vi "Handle Last Ack Core.vi"(4 "error in (no error)":errorcluster, 6 "Last Ack":refnum<class "Last Ack.lvclass">, 7 "Application in":refnum<class "Application.lvclass">) -> (0 "error out":errorcluster, 3 "Application out":refnum<class "Application.lvclass">)   [LabVIEW 2022 SP3, in "Application.lvlib" / "Application.lvclass"]
doc: "(<B>Filename</B>: Actor Framework.lvlib:Actor.lvclass:Handle Last Ack Core.vi)\n\nDefines how the caller actor responds to the Last Ack message from a nested actor. The Last Ack message is the final message a nested actor sends to its caller before it shuts down. The message contains information about the final state of the nested actor.\n\nBy default, this method does nothing except return any error the nested actor sent. A descendant class may override this method to define behavior."
uses:
  Application.lvclass
  <vilib>/ActorFramework/LastAck/Last Ack.lvclass
  C:/Program Files/National Instruments/LabVIEW 2022/vi.lib/ActorFramework/Actor/Actor.lvclass
  <vilib>/ActorFramework/LastAck/Last Ack.lvclass/Last Ack.ctl
  <vilib>/ActorFramework/Actor/Actor.lvclass/Actor.ctl
  <vilib>/ActorFramework/Message Enqueuer/Message Enqueuer.lvclass/Message Enqueuer.ctl
  <vilib>/ActorFramework/Message Enqueuer/Init from Existing Queue.vi
  <vilib>/ActorFramework/Message Enqueuer/Enqueue.vi
  <vilib>/ActorFramework/Stop Msg/Stop Msg.lvclass
  C:/Program Files/National Instruments/LabVIEW 2022/vi.lib/ActorFramework/Message/Message.lvclass
  <vilib>/ActorFramework/Message Priority Queue/Priority Enqueue.vi
  <vilib>/ActorFramework/Message Enqueuer/Message Enqueuer.lvclass
  Application.lvclass/Application.ctl
  <vilib>/ActorFramework/Actor/Actor.lvclass
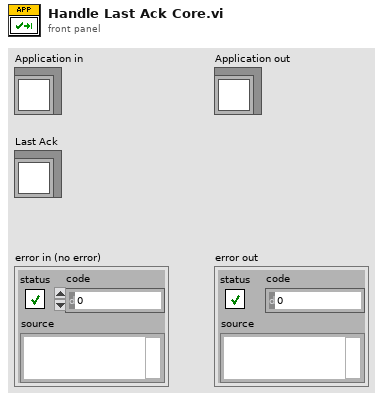
[diagram p1: front panel]
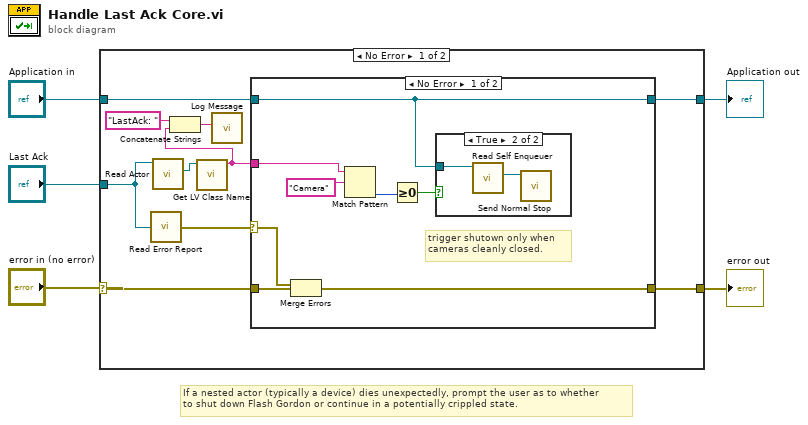
[diagram p0: block diagram]
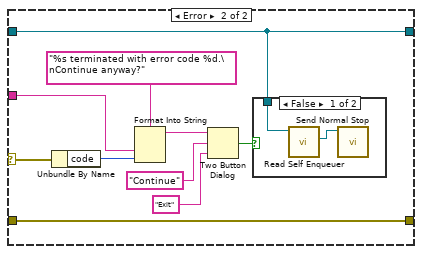
[diagram p3: hidden frame]
diagram:
  # "If a nested actor (typically a device) dies unexpectedly, prompt the user as to whether\nto shut down Flash Gordon or continue in a potentially crippled state."
  n1 = case shown="No Error" "error in (no error)" {
    selector: "error in (no error)" -> [w12 w38]
    tunnel: [w13 w38] -> w5
    tunnel: [w10 w39] -> w4
    tunnel: "Application in" -> [w11 w39]
    tunnel: "Last Ack" -> [w15 _]
    frame No Error {
      n2 = call <vilib>:"Read Error Report.vi"("Last Ack"=w15) -> ("error report"=w14:errorcluster)
      n3 = call <vilib>:"Read Actor.vi"("Last Ack"=w15) -> ("Actor"=w9:refnum<class "Actor.lvclass">)  [unwired: 10 in]
      n4 = call <vilib>:"Get LV Class Name.vi"("object"=w9) -> ("class name"=w7:string)  [unwired: 9 in, 1 out]
      n5 = Concatenate Strings("LastAck: " ("string"), w7) -> (w8:string)
      n6 = call "Log Message.vi"("input"=w8) -> ()  [unwired: 9 in, 2 out]
      n7 = case shown="No Error" w14 {
        selector: w14 -> [w17 w31]
        tunnel: [w16 w28] -> w13
        tunnel: w12 -> [w18 w28]
        tunnel: w11 -> [w20 w30]
        tunnel: [w20 w30] -> w10
        tunnel: w7 -> [w19 w26]
        frame No Error {
          # "trigger shutown only when\ncameras cleanly closed."
          n8 = Merge Errors(w17, w18) -> (w16:errorcluster)
          n9 = Match Pattern(string=w19, regular expression="Camera") -> (offset past match=w22:i32)  [unwired: 1 in, 3 out]
          n10 = Greater Or Equal To 0?(x=w22) -> (x >= 0?=w21:bool)
          n11 = case shown="True" w21 {
            tunnel: w20 -> [_ w24]
            frame False {
            }
            frame True {
              n12 = call <vilib>:"Read Self Enqueuer.vi"("Actor"=w24) -> ("Self Enqueuer"=w25:refnum<class "Message Enqueuer.lvclass">)  [unwired: 10 in]
              n13 = call <vilib>:"Send Normal Stop.vi"("Message Enqueuer"=w25) -> ()  [unwired: 10 in, 1 out]
            }
          }
        }
        frame Error {
          n14 = Unbundle By Name(w31) -> ("code"=w35:i32)
          n15 = Format Into String(format string="%s terminated with error code %d.\nContinue anyway?" ("string"), w26, w35) -> (resulting string=w33:string)  [unwired: 2 in, 1 out]
          n16 = Two Button Dialog(message=w33, 1:"Exit" ("F button name (\"Cancel\")"), 2:"Continue" ("T button name (\"OK\")")) -> (T button?=w29:bool)
          n17 = case shown="False" w29 {
            tunnel: w30 -> [w36 _]
            frame False {
              n18 = call <vilib>:"Read Self Enqueuer.vi"("Actor"=w36) -> ("Self Enqueuer"=w37:refnum<class "Message Enqueuer.lvclass">)  [unwired: 10 in]
              n19 = call <vilib>:"Send Normal Stop.vi"("Message Enqueuer"=w37) -> ()  [unwired: 10 in, 1 out]
            }
            frame True {
            }
          }
        }
      }
    }
    frame Error {
    }
  }
  "Application out" <- w4
  "error out" <- w5
